vi "芯片ID.vi"() -> ()   [LabVIEW 2013]
uses:
  <vilib>/Utility/error.llb/whitespace.ctl
panel:
  out "元素":string
  out "Row":i32
  out "设备号字符":string
  in  "合格":bool
  in  "设备号":u16(ring)=1 items=["00", "01", "02", "03", "04", "05", "06", "07", "08", "09", "10", "11", "12", "13", "14"]
  in  "写入质量数据":bool
  in  "总成ID":string
  in  "Table 2":string[][](table) caption="合格查询"
  in  "合格查询":bool
  out "error out":errorcluster
  in  "芯片查询":bool
  out "Table":string[][](table) caption="芯片"
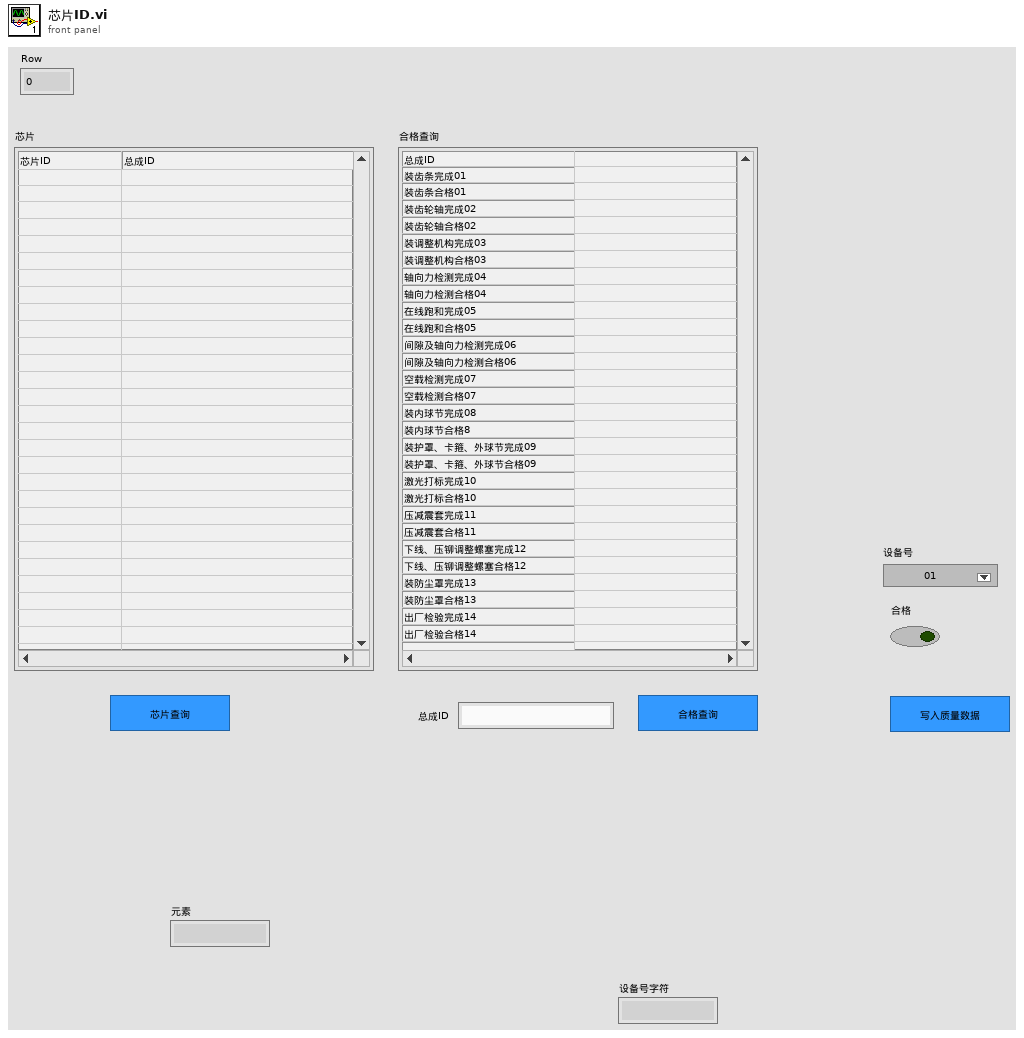
[diagram p1: front panel]
types:
  T1 = typedef "LVRowAndColumnTypeDef.ctl" = cluster{"Row":i32, "Column":i32}
  T2 = typedef "whitespace.ctl" = u16
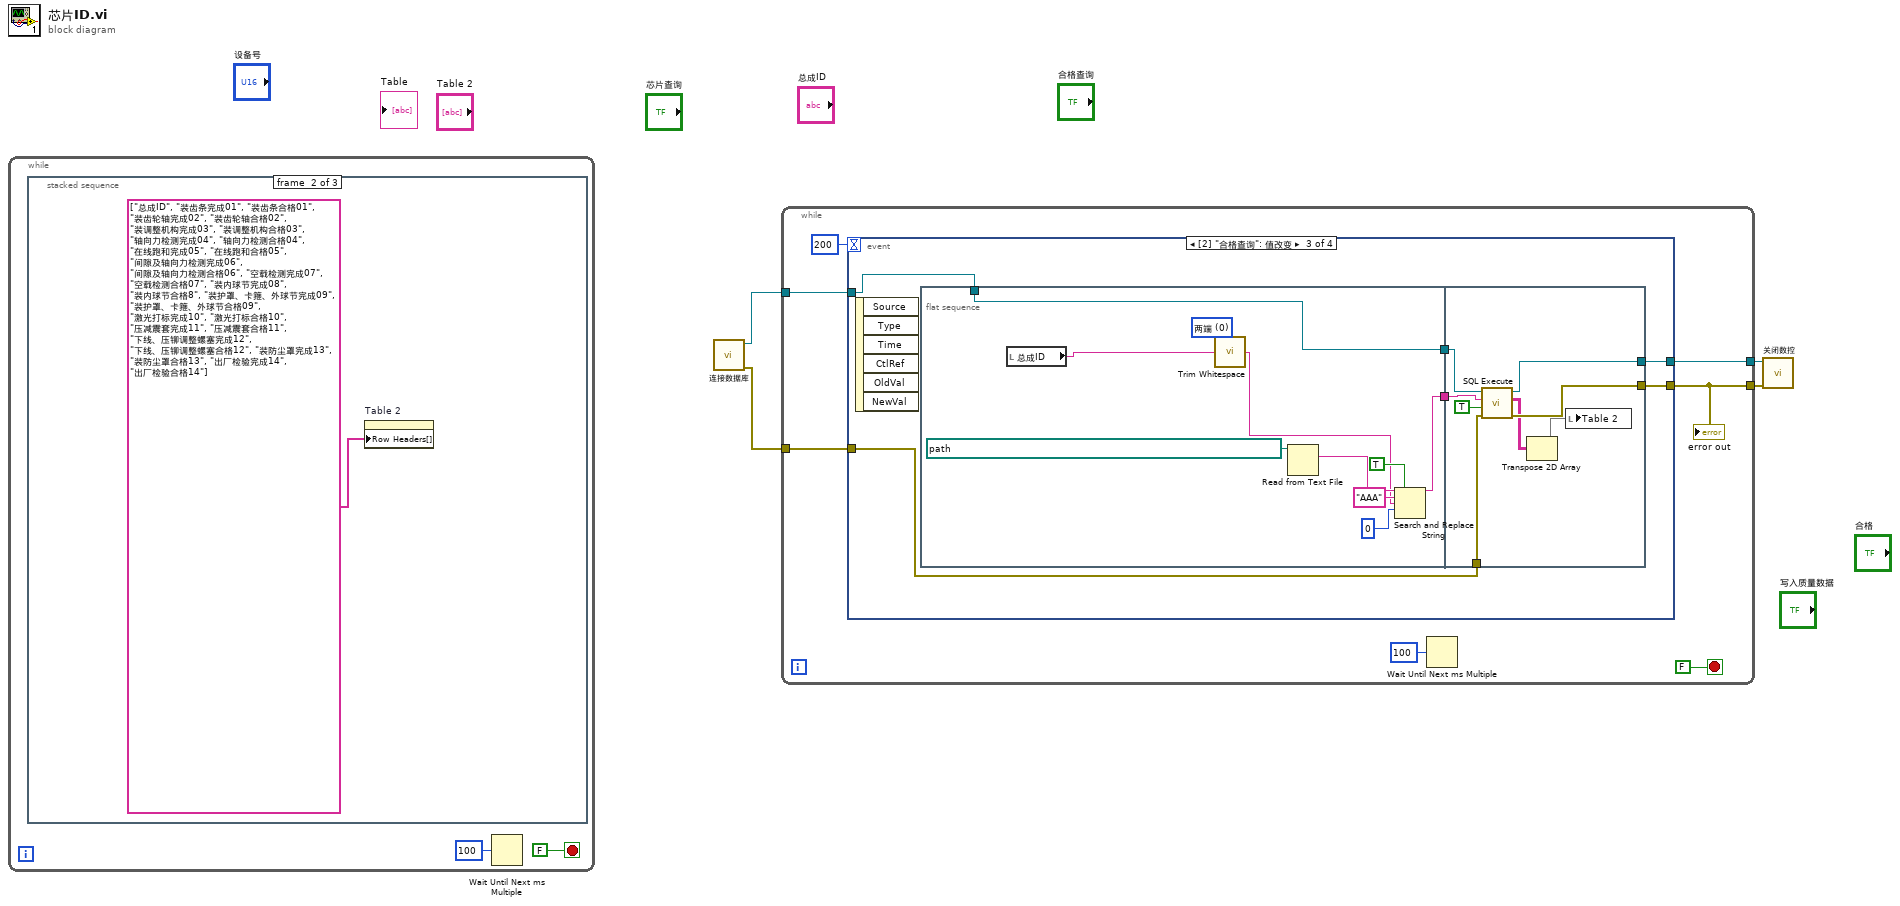
[diagram p0: block diagram]
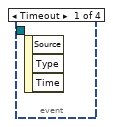
[diagram p2: hidden frame]
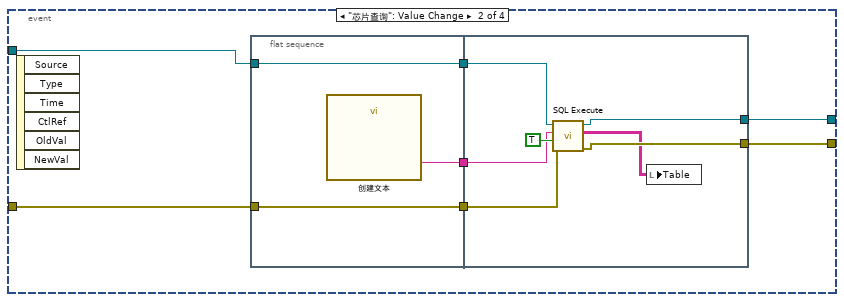
[diagram p3: hidden frame]
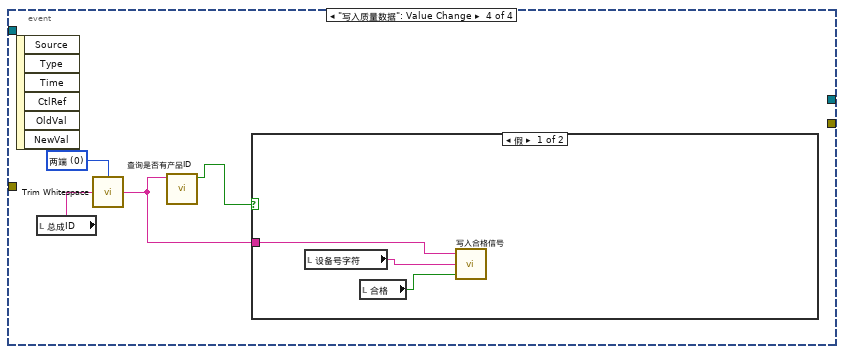
[diagram p4: hidden frame]
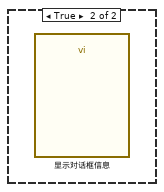
[diagram p5: hidden frame]
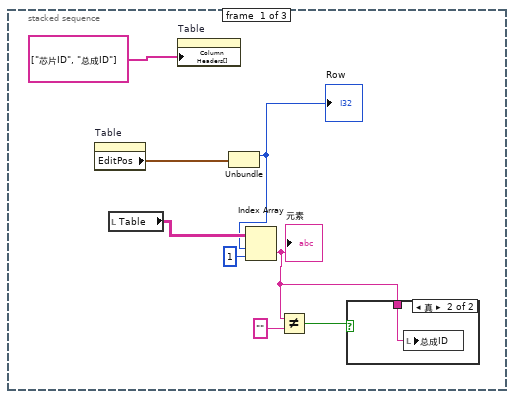
[diagram p6: hidden frame]
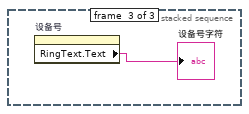
[diagram p8: hidden frame]
diagram:
  n1 = while {
    stop <- FALSE stop-if-true
    n2 = stacked-sequence {
      frame #0 {
        n3 = property on="Table" class="Tbl (严格)"() -> ("EditPos"=w13:T1)  [unwired: 2 in, 2 out]
        n4 = local read "Table"() -> (w12:string[][])
        n5 = property on="Table" class="Tbl (严格)"("Column Headers[]"=string[] ["芯片ID", "总成ID"] ("行首字符串[]")) -> ()  [unwired: 2 in, 2 out]
        n6 = Unbundle(w13) -> ("Row"=w10:i32)  [unwired: 1 out]
        "Row" <- w10
        n7 = Index Array(array=w12, index (row)=w10, index (col)=1 ("禁用的索引 (列)")) -> (element=w7:string)
        "元素" <- w7
        n8 = Not Equal?(x=w7, y="") -> (x != y?=w8:bool)
        n9 = case shown="真" w8 {
          tunnel: w7 -> [_ w15]
          frame False {
          }
          frame True {
            n10 = local write "总成ID"(w15) -> ()
          }
        }
      }
      frame #1 {
        n11 = property on="Table 2" class="Tbl (严格)"("Row Headers[]"=string[] ["总成ID", "装齿条完成01", "装齿条合格01", "装齿轮轴完成02", "装齿轮轴合格02", "装调整机构完成03", "装调整机构合格03", "轴向力检测完成04", "轴向力检测合格04", "在线跑和完成05", "在线跑和合格05", "间隙及轴向力检测完成06", "间隙及轴向力检测合格06", "空载检测完成07", "空载检测合格07", "装内球节完成08", "装内球节合格8", "装护罩、卡箍、外球节完成09", "装护罩、卡箍、外球节合格09", "激光打标完成10", "激光打标合格10", "压减震套完成11", "压减震套合格11", "下线、压铆调整螺塞完成12", "下线、压铆调整螺塞合格12", "装防尘罩完成13", "装防尘罩合格13", "出厂检验完成14", "出厂检验合格14"] ("行首字符串[]")) -> ()  [unwired: 2 in, 2 out]
      }
      frame #2 {
        n12 = property on="设备号" class="Ring (严格)"() -> ("RingText.Text"=→"设备号字符":string)  [unwired: 2 in, 2 out]
      }
    }
    n13 = Wait Until Next ms Multiple(millisecond multiple=u32 100 ("毫秒倍数")) -> ()  [unwired: 1 out]
  }
  n14 = call "连接数据库.vi"() -> ("error out"=w2:errorcluster, "ADODB._Connection Out"=w4:refnum<k7>)  [unwired: 10 in]
  n15 = while {
    tunnel: w4 -> [w21]
    tunnel: [w20] -> w3
    tunnel: w2 -> [w19]
    tunnel: [w18] -> w1
    stop <- FALSE stop-if-true
    n16 = event shown="[2] \"合格查询\": 值改变" {
      selector: _ -> [_ _ _ _]
      dyn-events: _ -> [_ _ _ _]
      timeout: 200 -> [_ _ _ _]
      tunnel: w21 -> [_ w29 w47 _]
      tunnel: [_ w28 w45 _] -> w20
      tunnel: w19 -> [_ w26 w46 _]
      tunnel: [_ w25 w44 _] -> w18
      event Timeout {
        n17 = event-data() -> ()  [unwired: 1 in, 3 out]
      }
      event "芯片查询": Value Change {
        n18 = event-data() -> ()  [unwired: 1 in, 6 out]
        n19 = flat-sequence {
          tunnel: [w34] -> w31
          tunnel: [w33] -> w30
          tunnel: w29 -> [w33]
          tunnel: [w32] -> w27
          tunnel: w26 -> [w32]
          tunnel: w31 -> [w40]
          tunnel: w30 -> [w39]
          tunnel: [w38] -> w28
          tunnel: w27 -> [w37]
          tunnel: [w36] -> w25
          frame #0 {
            n20 = call "创建文本"() -> ("Result"=w34:string)  [unwired: 14 in, 1 out]
          }
          frame #1 {
            n21 = call "SQL Execute.vi"("error in (no error)"=w37, "Return Data (T)"=TRUE, "Command Text"=w40, "ADODB._Connection In"=w39) -> ("error out"=w36:errorcluster, "Data"=w35:string[][], "ADODB._Connection Out"=w38:refnum<k7>)  [unwired: 4 in, 1 out]
            n22 = local write "Table"(w35) -> ()
          }
        }
      }
      event "合格查询": Value Change {
        n23 = event-data() -> ()  [unwired: 1 in, 6 out]
        n24 = flat-sequence {
          tunnel: w47 -> [w50]
          tunnel: [w50] -> w43
          tunnel: [w48] -> w42
          tunnel: w46 -> [w64]
          tunnel: [w63] -> w45
          tunnel: [w62] -> w44
          tunnel: w43 -> [w61]
          tunnel: w42 -> [w60]
          frame #0 {
            w57 = T2 0 items=["两端", "字符串首端", "字符串末端"] ("location (both)")
            n25 = local read "总成ID"() -> (w51:string)
            n26 = call <vilib>:"Trim Whitespace.vi"("string"=w51, "location (both)"=w57) -> ("trimmed string"=w52:string)
            n27 = Read from Text File(file (use dialog)=path "F:/Q14070/Q14070生产管理系统/子VI/产品ID质量数据查询.txt" ("文件（使用对话框）")) -> (text=w54:string)  [unwired: 3 in, 3 out]
            n28 = Search and Replace String(replace all?=TRUE ("替换全部？(F)"), input string=w54, search string="AAA" ("搜索字符串"), replace string=w52, offset=0 ("偏移量(0)")) -> (result string=w48:string)  [unwired: 3 in, 3 out]
          }
          frame #1 {
            n29 = call "SQL Execute.vi"("error in (no error)"=w64, "Return Data (T)"=TRUE, "Command Text"=w60, "ADODB._Connection In"=w61) -> ("error out"=w62:errorcluster, "Data"=w59:string[][], "ADODB._Connection Out"=w63:refnum<k7>)  [unwired: 4 in, 1 out]
            n30 = Transpose 2D Array(2D array=w59) -> (transposed array=w58:string[][])
            n31 = local write "Table 2"(w58) -> ()
          }
        }
      }
      event "写入质量数据": Value Change {
        w67 = T2 0 items=["两端", "字符串首端", "字符串末端"] ("location (both)")
        n32 = event-data() -> ()  [unwired: 1 in, 6 out]
        n33 = local read "总成ID"() -> (w66:string)
        n34 = call <vilib>:"Trim Whitespace.vi"("string"=w66, "location (both)"=w67) -> ("trimmed string"=w69:string)
        n35 = call "查询是否有产品ID.vi"("转向器总成ID"=w69) -> ("无重号"=w68:bool)  [unwired: 9 in, 1 out]
        n36 = case shown="假" w68 {
          tunnel: w69 -> [w72 _]
          frame False {
            n37 = local read "设备号字符"() -> (w71:string)
            n38 = local read "合格"() -> (w70:bool)
            n39 = call "写入合格信号.vi"("信号"=w70, "设备号"=w71, "产品ID"=w72) -> ()  [unwired: 2 in]
          }
          frame True {
            n40 = call "显示对话框信息"() -> ()  [unwired: 10 in, 2 out]
          }
        }
      }
    }
    "error out" <- w18
    n41 = Wait Until Next ms Multiple(millisecond multiple=u32 100 ("毫秒倍数")) -> ()  [unwired: 1 out]
  }
  n42 = call "关闭数控.vi"("error in (no error)"=w1, "ADODB._Connection In"=w3) -> ()  [unwired: 9 in, 1 out]
